vi "Sync_Afterwards.vi"(2 "Analogue Data":dbl[][](array[numeric]) format="%.3f", 4 "LDA Data":dbl[][](array[numeric]) format="%.3f") -> (0 "Eng Values":dbl[][](array[numeric]) format="%.2f")   [LabVIEW 2010]
uses:
  Globals/LDA_meas_global_1.vi
  Globals/Meas_global.vi
  Globals/Dynamic_call_global.ph.vi
panel:
  out "Array":string[](array[string])
  out "Delay (ms)":dbl=13.0 format="%.2f"
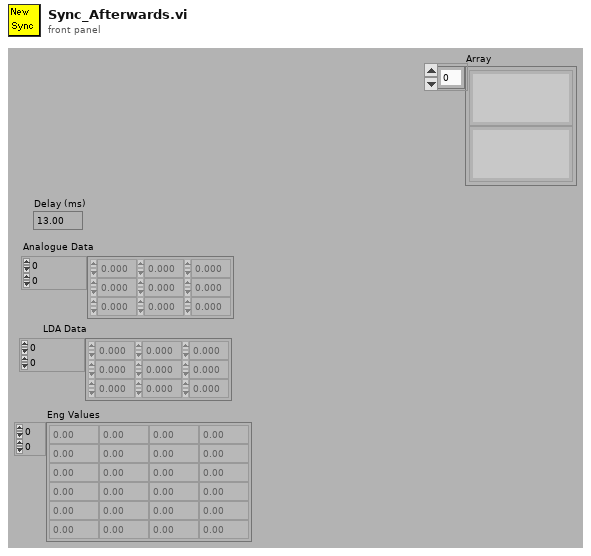
[diagram p1: front panel]
types:
  T1 = typedef "Analysis_info_cluster.ctl" = cluster{"Colour":u32, "Inst type":T2, "Inst name":string, "Symbol":string, "Code name":string, "Extra Info":string, "Inst Array":T3, "Index":i32, "Voltage Index":i32, "Extra Titles":string[], "Extra Values":string[]}
  T2 = typedef "Inst_type.ctl" = enum16{"Propeller anemometer", "Raw voltage", "Pressure Transducer", "Pitot-static tube", "Preston tube", "Hot wire", "Cross wire 1", "Cross wire 2", "Generic Linear", "Generic Polynomial", "Generic BackPoly", "Fast FID", "Thermocouple", "Cold wire", "Pulsed Wire", "LDA Vel", "LDA Tran time", "LDA Arr time"}
  T3 = typedef "Instrument_Array.ctl" = enum16{"PWA", "LDA", "Analogue"}
  T4 = typedef "Analysis_type_cluster.ctl" = cluster{"Analysis type":T5, "Indicies":i32[], "Name":string, "Inst Array":T3, "Info index":i32}
  T5 = typedef "Analysis_type_Enum.ctl" = enum16{"Slow Response", "Fast Response", "Weighted Fast Response", "Fast FID", "Weighted Fast FID", "Cross Wire", "Weighted Cross Wire", "Weighted LDA"}
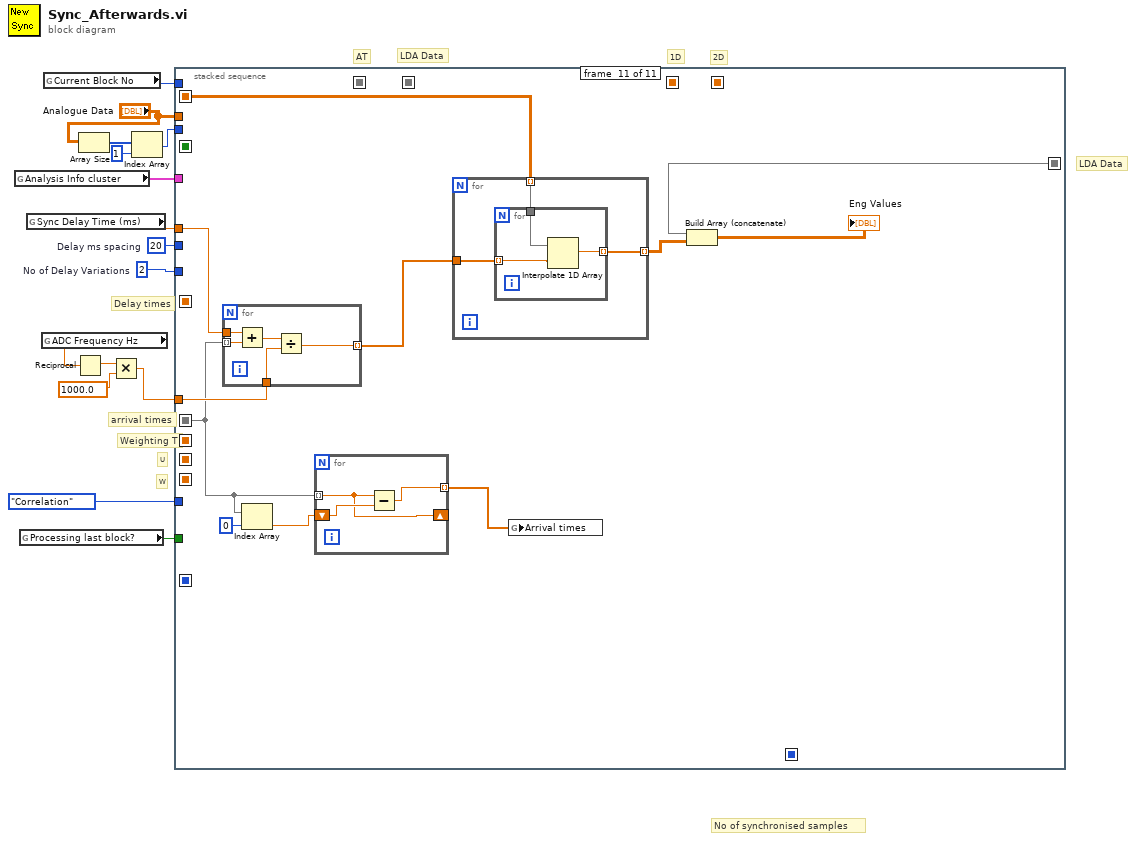
[diagram p0: block diagram]
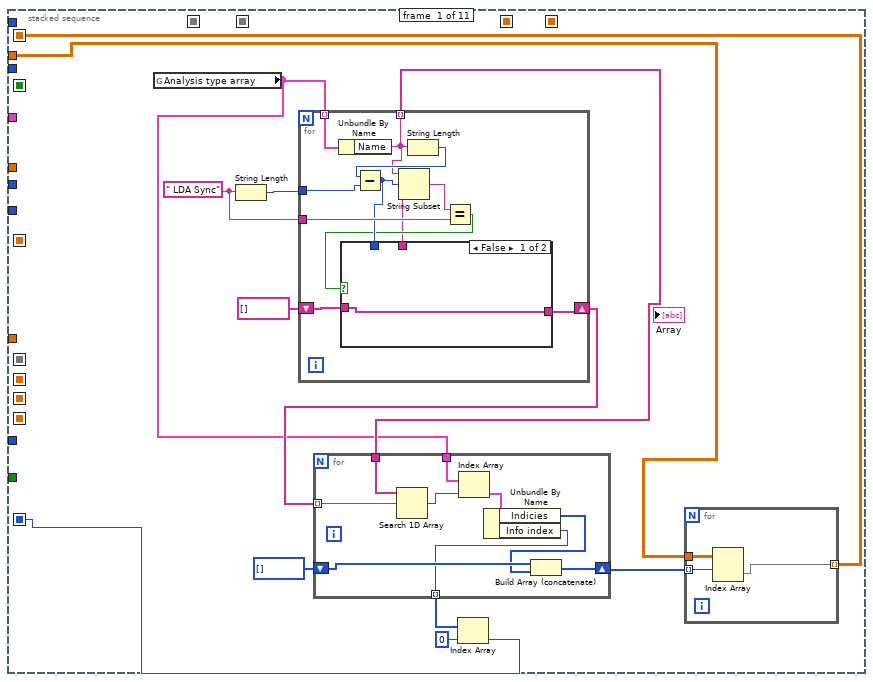
[diagram p2: hidden frame]
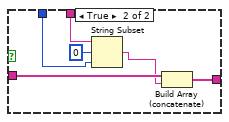
[diagram p3: hidden frame]
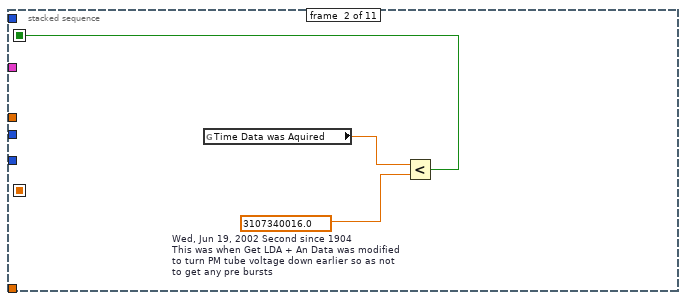
[diagram p4: hidden frame]
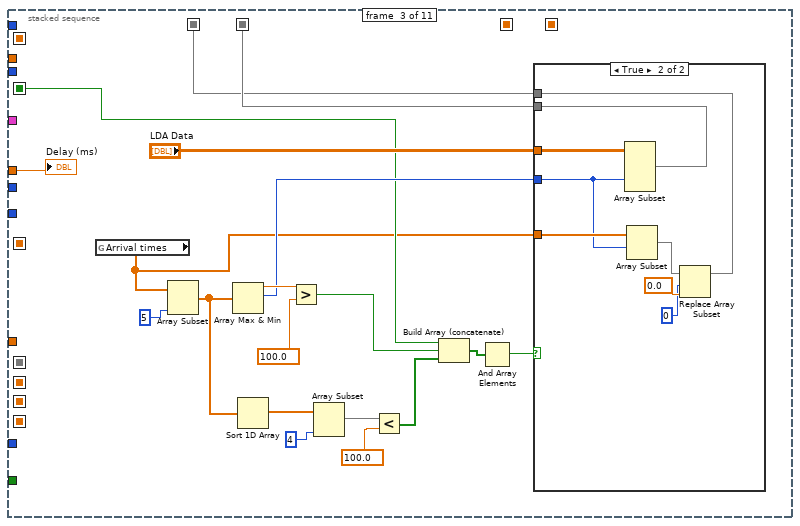
[diagram p5: hidden frame]
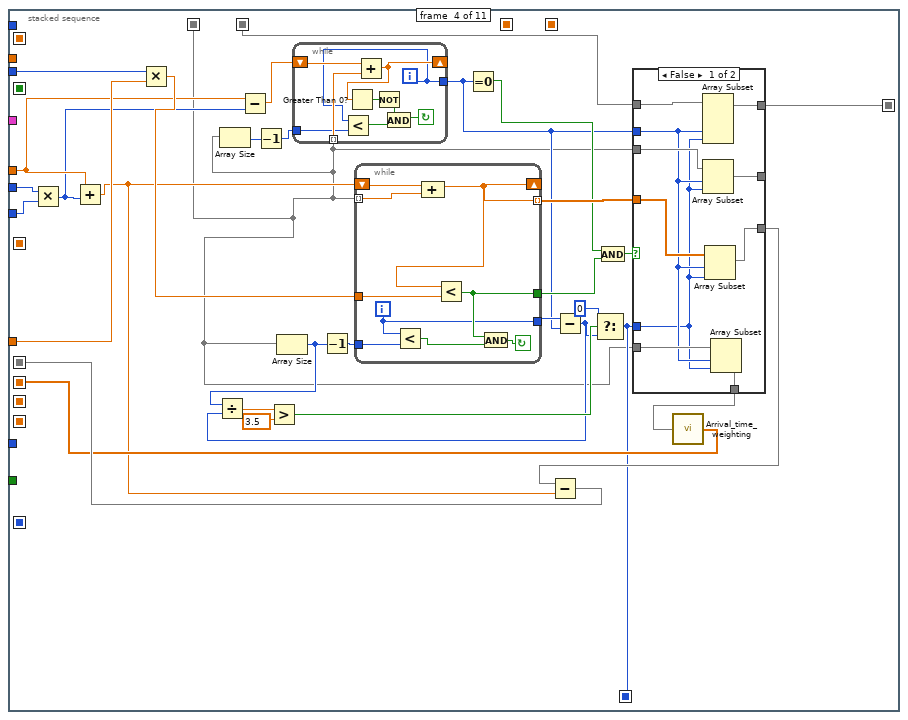
[diagram p7: hidden frame]
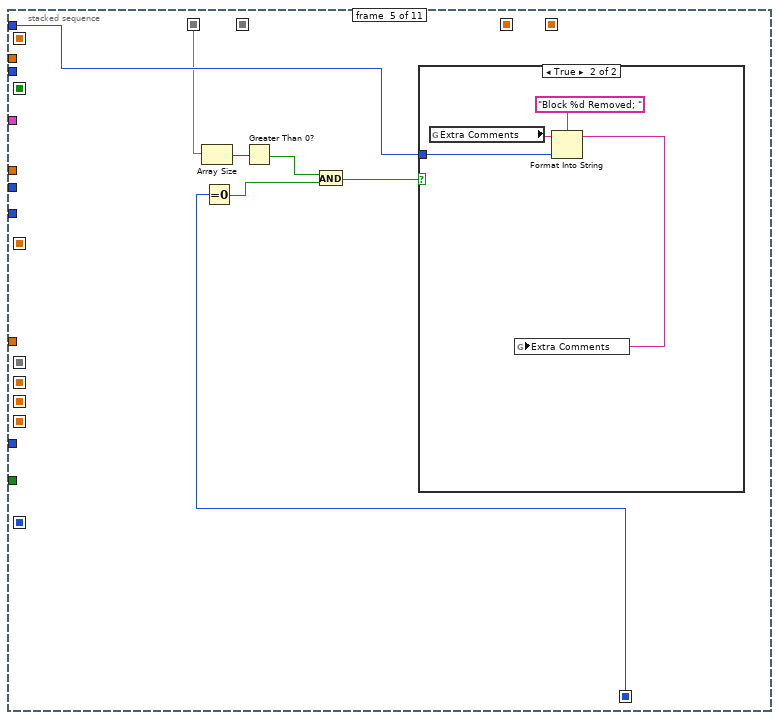
[diagram p9: hidden frame]
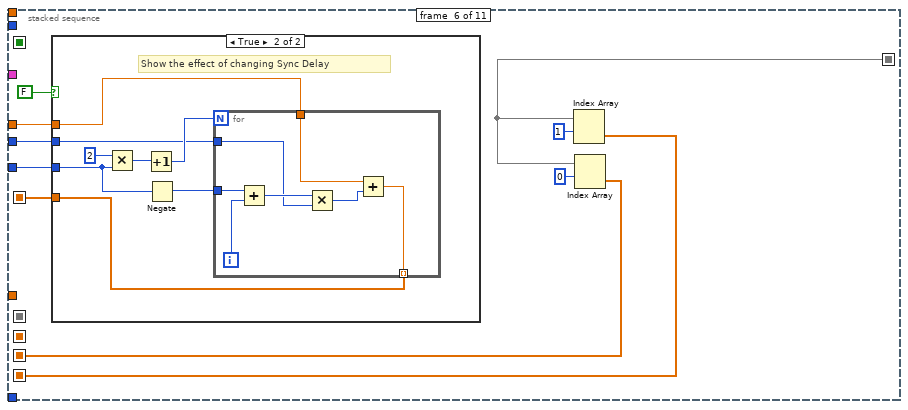
[diagram p11: hidden frame]
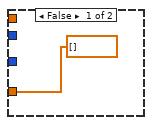
[diagram p12: hidden frame]
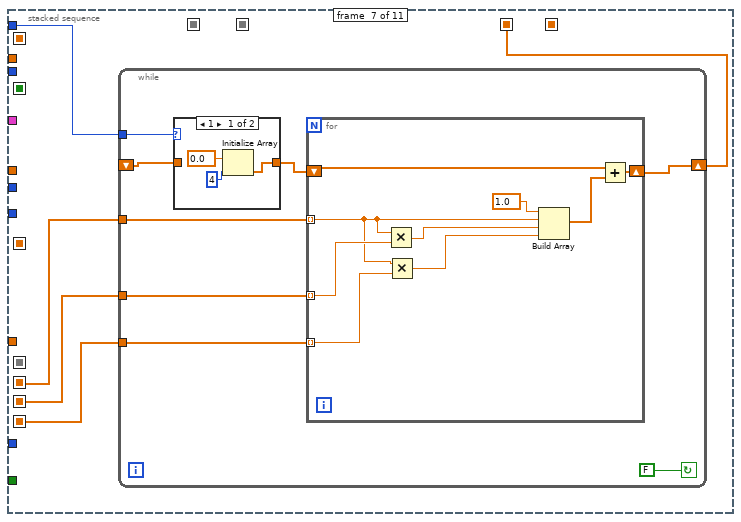
[diagram p13: hidden frame]
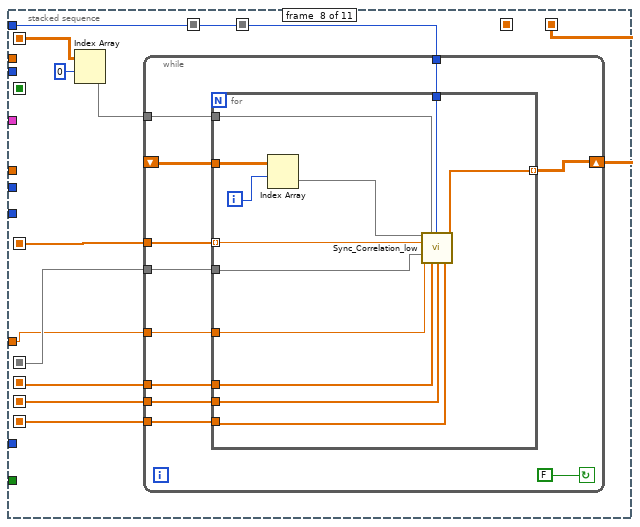
[diagram p15: hidden frame]
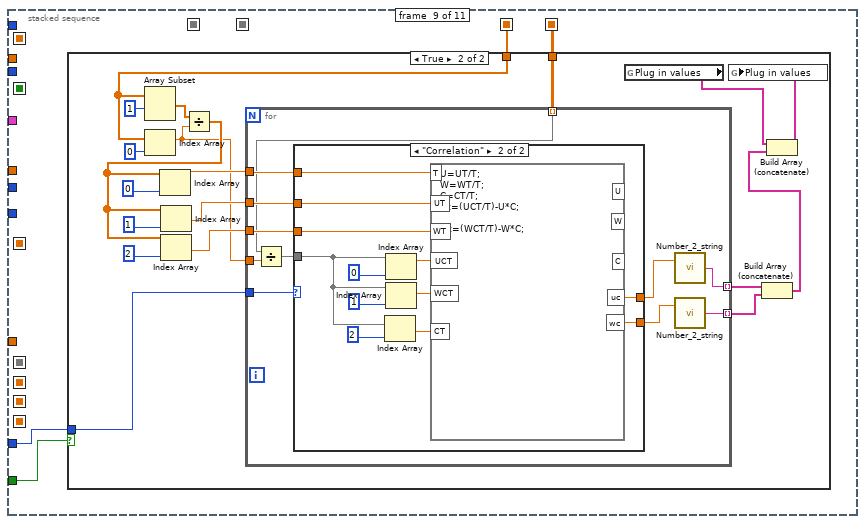
[diagram p16: hidden frame]
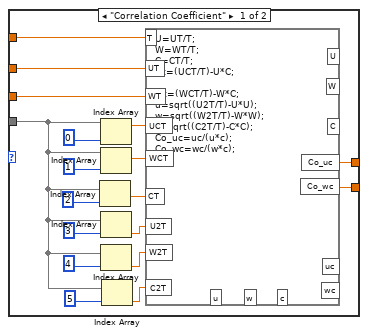
[diagram p18: hidden frame]
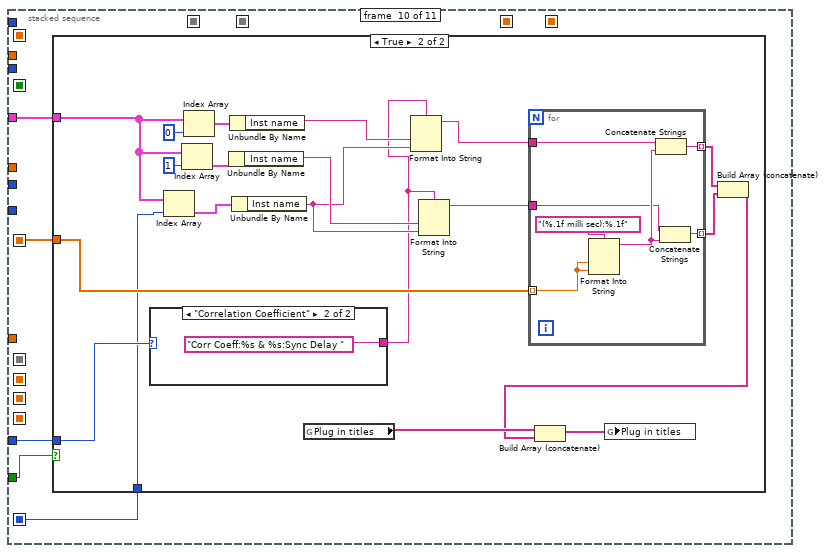
[diagram p19: hidden frame]
diagram:
  w3 = 20  # Delay ms spacing
  w15 = 2  # No of Delay Variations
  # "No of synchronised samples"
  # "AT"
  # "LDA Data"
  # "Delay times"
  # "1D"
  # "2D"
  # "W"
  # "U"
  # "Weighting T"
  # "arrival times"
  # "LDA Data"
  n1 = global read "Meas_global.vi" "Analysis Info cluster"() -> (w1:T1[])
  n2 = global read "Meas_global.vi" "Processing last block?"() -> (w13:bool)
  n3 = global read "LDA_meas_global_1.vi" "Sync Delay Time (ms)"() -> (w8:dbl)
  n4 = global read "LDA_meas_global_1.vi" "ADC Frequency Hz"() -> (w11:dbl)
  n5 = global read "Meas_global.vi" "Current Block No"() -> (w14:i32)
  n6 = Reciprocal(x=w11) -> (1/x=w12:dbl)
  n7 = Array Size(array="Analogue Data") -> (size(s)=w6:i32[])
  n8 = Multiply(x=w12, y=1000.0) -> (x*y=w9:dbl)
  n9 = Index Array(array=w6, index=1 ("Index")) -> (element=w4:i32)
  n10 = stacked-sequence {
    seq-local: [_ _ _ w119 _ _ _ _ _ _ _] -> [_ _ _ _ _ w170 _ _ _ _ w357]
    seq-local: [_ _ _ w116 _ _ _ _ _ _ _] -> [_ _ _ _ _ _ _ w222 _ _ w351]
    seq-local: [_ _ _ w114 _ _ _ _ _ _ _] -> [_ _ _ _ _ _ w195 w223 _ _ _]
    seq-local: [_ _ _ _ _ w169 _ _ _ _ _] -> [_ _ _ _ _ _ w194 w225 _ _ _]
    seq-local: [_ _ _ _ _ w168 _ _ _ _ _] -> [_ _ _ _ _ _ w193 w224 _ _ _]
    seq-local: [_ _ _ _ _ _ _ w220 _ _ _] -> [_ _ _ _ _ _ _ _ w252 _ _]
    seq-local: [_ _ _ _ _ _ w191 _ _ _ _] -> [_ _ _ _ _ _ _ _ w253 _ _]
    seq-local: [_ _ _ _ _ w173 _ _ _ _ _] -> [_ _ _ _ _ _ _ w219 _ w318 _]
    seq-local: [_ _ w66 _ _ _ _ _ _ _ _] -> [_ _ _ w106 _ _ _ _ _ _ _]
    seq-local: [_ _ w65 _ _ _ _ _ _ _ _] -> [_ _ _ w92 w159 _ _ _ _ _ _]
    seq-local: [_ w59 _ _ _ _ _ _ _ _ _] -> [_ _ w62 _ _ _ _ _ _ _ _]
    seq-local: [_ _ _ w96 _ _ _ _ _ _ _] -> [_ _ _ _ w158 _ _ _ _ _ _]
    seq-local: [w17 _ _ _ _ _ _ _ _ _ _] -> [_ _ _ _ _ _ _ _ _ w315 _]
    seq-local: [w16 _ _ _ _ _ _ _ _ _ _] -> [_ _ _ _ _ _ _ w217 _ _ w354]
    tunnel: "Analogue Data" -> [w20 _ _ _ _ _ _ _ _ _ _]
    tunnel: w8 -> [_ _ w63 w108 _ w167 _ _ _ _ w353]
    tunnel: w15 -> [_ _ _ w94 _ w174 _ _ _ _ _]
    tunnel: w14 -> [_ _ _ _ w160 _ w192 w221 _ _ _]
    tunnel: w13 -> [_ _ _ _ _ _ _ _ w254 w319 _]
    tunnel: w9 -> [_ _ _ w113 _ _ _ w218 _ _ w359]
    tunnel: w4 -> [_ _ _ w98 _ _ _ _ _ _ _]
    tunnel: w3 -> [_ _ _ w95 _ w166 _ _ _ _ _]
    tunnel: enum16{"Correlation", "Correlation Coefficient"}."Correlation" -> [_ _ _ _ _ _ _ _ w251 w317 _]
    tunnel: w1 -> [_ _ _ _ _ _ _ _ _ w316 _]
    frame #0 {
      w27 = " LDA Sync" ("Substring")
      n11 = global read "Meas_global.vi" "Analysis type array"() -> (w23:T4[])
      n12 = String Length(string=w27) -> (length=w26:i32)
      n13 = for {
        tunnel: w23 -> [w50] mode=indexing
        tunnel: w26 -> [w48]
        tunnel: w27 -> [w46]
        shift-right: [w42] -> w24
        shift-left: string[] [] -> [w43]
        tunnel: [w41] -> w25 mode=indexing
        n14 = Unbundle By Name(w50) -> ("Name"=w41:string)
        n15 = String Length(string=w41) -> (length=w49:i32)
        n16 = Subtract(x=w49, y=w48) -> (x-y=w45:i32)
        n17 = String Subset(string=w41, offset (0)=w45) -> (substring=w47:string)  [unwired: 1 out]
        n18 = Equal?(x=w47, y=w46) -> (x = y?=w44:bool)
        n19 = case shown="False" w44 {
          tunnel: w41 -> [_ w57]
          tunnel: w45 -> [_ w55]
          tunnel: w43 -> [w51 w54]
          tunnel: [w51 w52] -> w42
          frame False {
          }
          frame True {
            n20 = String Subset(string=w57, offset (0)=0, length (rest)=w55) -> (substring=w53:string)
            n21 = Build Array (concatenate)(w54, w53) -> (w52:string[])
          }
        }
      }
      n22 = for {
        tunnel: w25 -> [w40]
        tunnel: w24 -> [w39] mode=indexing
        tunnel: w23 -> [w38]
        shift-right: [w34] -> w21
        shift-left: i32[] [] -> [w36]
        tunnel: [w32] -> w19 mode=indexing
        n23 = Search 1D Array(1D array=w40, element=w39) -> (index of element=w33:i32)  [unwired: 1 out]
        n24 = Index Array(array=w38, index=w33) -> (element=w37:T4)
        n25 = Unbundle By Name(w37) -> ("Indicies"=w35:i32[], "Info index"=w32:i32)
        n26 = Build Array (concatenate)(w36, w35) -> (w34:i32[])
      }
      n27 = Index Array(array=w19, index=0) -> (element=w17:i32)
      n28 = for {
        tunnel: w21 -> [w31] mode=indexing
        tunnel: w20 -> [w30]
        tunnel: [w29] -> w16 mode=indexing
        n29 = Index Array(array=w30, index (row)=w31) -> (element=w29:dbl[])  [unwired: 1 in]
      }
    }
    frame #1 {
      w60 = 3107340016.0  # Wed, Jun 19, 2002 Second since 1904 This was when Get LDA + An Data was modified to turn PM tube voltage down earlier so as not to get any pre bursts
      n30 = global read "Meas_global.vi" "Time Data was Aquired"() -> (w58:dbl)
      n31 = Less?(x=w58, y=w60) -> (x < y?=w59:bool)
    }
    frame #2 {
      n32 = global read "LDA_meas_global_1.vi" "Arrival times"() -> (w61:dbl[])
      n33 = Array Subset(array=w61, length=5 ("Array Length")) -> (w76:dbl[])  [unwired: 1 in]
      n34 = Array Max & Min(array=w76) -> (max value=w78:dbl, max index (indices)=w68:i32)  [unwired: 2 out]
      n35 = Sort 1D Array(array=w76) -> (sorted array=w74:dbl[])
      n36 = Greater?(x=w78, y=100.0) -> (0:w70:bool)
      n37 = Array Subset(array=w74, length=4 ("Array Length")) -> (w73:dbl[])  [unwired: 1 in]
      n38 = Less?(x=w73, y=100.0) -> (x < y?=w71:bool[])
      n39 = Build Array (concatenate)(w62, w70, w71) -> (w69:bool[])
      n40 = And Array Elements(Boolean array=w69) -> (logical AND=w64:bool)
      n41 = case shown="True" w64 {
        tunnel: w68 -> [_ w82]
        tunnel: "LDA Data" -> [w80 w89]
        tunnel: [w80 w88] -> w66
        tunnel: w61 -> [w81 w87]
        tunnel: [w81 w83] -> w65
        frame False {
        }
        frame True {
          n42 = Array Subset(array=w89, index (col)=w82) -> (w88:dbl[][])  [unwired: 3 in]
          n43 = Array Subset(array=w87, index=w82) -> (w86:dbl[])  [unwired: 1 in]
          n44 = Replace Array Subset(array=w86, new element=0.0 ("Element Data"), index=0 ("Index")) -> (w83:dbl[])
        }
      }
      "Delay (ms)" <- w63
    }
    frame #3 {
      n45 = Multiply(x=w95, y=w94) -> (x*y=w93:i32)
      n46 = Add(x=w108, y=w93) -> (x+y=w112:dbl)
      n47 = Multiply(x=w98, y=w113) -> (x*y=w120:dbl)
      n48 = Array Size(array=w92) -> (size(s)=w91:i32)
      n49 = Subtract(x=w108, y=w93) -> (x-y=w107:dbl)
      n50 = Decrement(x=w91) -> (x-1=w90:i32)
      n51 = Array Size(array=w92) -> (size(s)=w101:i32)
      n52 = while {
        tunnel: [w132] -> w104
        tunnel: w92 -> [w134] mode=indexing
        shift-left: w107 -> [w139]
        shift-right: [w138] -> _
        tunnel: w90 -> [w131]
        i -> [w132]
        stop <- w135 continue-if-true
        n53 = Less?(x=w132, y=w131) -> (x < y?=w133:bool)
        n54 = Add(x=w139, y=w134) -> (x+y=w138:dbl)
        n55 = Greater Than 0?(x=w138) -> (x > 0?=w137:bool)
        n56 = Not(x=w137) -> (.not. x?=w136:bool)
        n57 = And(x=w136, y=w133) -> (x .and. y?=w135:bool)
      }
      n58 = Decrement(x=w101) -> (x-1=w121:i32)
      n59 = while {
        tunnel: [w122] -> w118 mode=indexing
        tunnel: [w123] -> w105
        tunnel: [w124] -> w111
        tunnel: w120 -> [w127]
        tunnel: w121 -> [w128]
        tunnel: w92 -> [w129] mode=indexing
        shift-left: w112 -> [w130]
        shift-right: [w122] -> _
        i -> [w123]
        stop <- w125 continue-if-true
        n60 = Less?(x=w123, y=w128) -> (x < y?=w126:bool)
        n61 = Compound Arithmetic op=ADD(w130, w129) -> (w122:dbl)
        n62 = Less?(x=w122, y=w127) -> (x < y?=w124:bool)
        n63 = And(x=w124, y=w126) -> (x .and. y?=w125:bool)
      }
      n64 = Equal To 0?(x=w104) -> (x = 0?=w110:bool)
      n65 = Subtract(x=w105, y=w104) -> (x-y=w97:i32)
      n66 = Divide(x=w101, y=w97) -> (x/y=w102:dbl)
      n67 = Greater?(x=w102, y=3.5) -> (0:w100:bool)
      n68 = Select(t=0, s=w100, f=w97) -> (s? t:f=w96:i32)
      n69 = And(x=w110, y=w111) -> (x .and. y?=w109:bool)
      n70 = case shown="False" w109 {
        tunnel: [w149 w152] -> w117
        tunnel: w96 -> [w141 _]
        tunnel: w106 -> [w148 w153]
        tunnel: [w147 w153] -> w119
        tunnel: w118 -> [w146 w152]
        tunnel: w92 -> [w145 w151]
        tunnel: [w144 w151] -> w115
        tunnel: w104 -> [w142 _]
        tunnel: w92 -> [w143 w150]
        tunnel: [w140 w150] -> _
        frame False {
          n71 = Array Subset(array=w148, index (col)=w142, length (col)=w141) -> (w147:dbl[][])  [unwired: 2 in]
          n72 = Array Subset(array=w143, index=w142, length=w141) -> (w140:dbl[])
          n73 = Array Subset(array=w146, index=w142, length=w141) -> (w149:dbl[])
          n74 = Array Subset(array=w145, index=w142, length=w141) -> (w144:dbl[])
        }
        frame True {
        }
      }
      n75 = Subtract(x=w117, y=w112) -> (x-y=w116:dbl[])
      n76 = call "Arrival_time_weighting.vi"("Arrival times"=w115) -> ("Weighting"=w114:dbl[])
    }
    frame #4 {
      n77 = Array Size(array=w159) -> (size(s)=w157:i32)
      n78 = Equal To 0?(x=w158) -> (x = 0?=w155:bool)
      n79 = Greater Than 0?(x=w157) -> (x > 0?=w156:bool)
      n80 = And(x=w156, y=w155) -> (x .and. y?=w154:bool)
      n81 = case shown="True" w154 {
        tunnel: w160 -> [_ w164]
        frame False {
        }
        frame True {
          n82 = global read "Meas_global.vi" "Extra Comments"() -> (w162:string)
          n83 = Format Into String(format string="Block %d Removed; " ("Format String"), initial string=w162, w164) -> (resulting string=w161:string)  [unwired: 1 in, 1 out]
          n84 = global write "Meas_global.vi" "Extra Comments"(w161) -> ()
        }
      }
    }
    frame #5 {
      n85 = case shown="True" FALSE {
        tunnel: w174 -> [_ w180]
        tunnel: [dbl[] [] w178] -> w173
        tunnel: w167 -> [_ w177]
        tunnel: w166 -> [_ w176]
        frame False {
        }
        frame True {
          # "Show the effect of changing Sync Delay"
          n86 = Multiply(x=2, y=w180) -> (x*y=w182:i32)
          n87 = Increment(x=w182) -> (x+1=w181:i32)
          n88 = Negate(x=w180) -> (-x=w179:i32)
          n89 = for {
            N: w181 -> [_]
            tunnel: w179 -> [w190]
            tunnel: w177 -> [w188]
            tunnel: [w187] -> w178 mode=indexing
            tunnel: w176 -> [w184]
            i -> [w189]
            n90 = Add(x=w190, y=w189) -> (x+y=w186:i32)
            n91 = Multiply(x=w186, y=w184) -> (x*y=w185:i32)
            n92 = Add(x=w188, y=w185) -> (x+y=w187:dbl)
          }
        }
      }
      n93 = Index Array(array=w170, index (row)=1 ("Index")) -> (element=w168:dbl[])  [unwired: 1 in]
      n94 = Index Array(array=w170, index (row)=0 ("Index")) -> (element=w169:dbl[])  [unwired: 1 in]
    }
    frame #6 {
      n95 = while {
        tunnel: w192 -> [w197]
        tunnel: w193 -> [w201]
        tunnel: w194 -> [w202]
        tunnel: w195 -> [w203]
        shift-left: _ -> [w199]
        shift-right: [w198] -> w191
        stop <- FALSE continue-if-true
        n96 = case shown="1" w197 {
          tunnel: [w204 w207] -> w200
          tunnel: w199 -> [_ w207]
          frame 1 {
            n97 = Initialize Array(0.0 ("Element Data"), 4 ("Dimension Size")) -> (w204:dbl[])
          }
          frame 2, Default {
          }
        }
        n98 = for {
          shift-right: [w215] -> w198
          shift-left: w200 -> [w216]
          tunnel: w203 -> [w211] mode=indexing
          tunnel: w202 -> [w214] mode=indexing
          tunnel: w201 -> [w210] mode=indexing
          n99 = Multiply(x=w211, y=w214) -> (x*y=w213:dbl)
          n100 = Multiply(x=w211, y=w210) -> (x*y=w209:dbl)
          n101 = Build Array(1.0 ("Input Element"), w211, w213, w209) -> (w208:dbl[])
          n102 = Add(x=w216, y=w208) -> (x+y=w215:dbl[])
        }
      }
    }
    frame #7 {
      n103 = Index Array(array=w217, index (row)=0 ("Index")) -> (element=w226:dbl[])  [unwired: 1 in]
      n104 = while {
        tunnel: w219 -> [w229]
        shift-left: _ -> [w231]
        shift-right: [w230] -> w220
        tunnel: w221 -> [w232]
        tunnel: w222 -> [w233]
        tunnel: w223 -> [w234]
        tunnel: w224 -> [w235]
        tunnel: w225 -> [w236]
        tunnel: w226 -> [w237]
        tunnel: w218 -> [w238]
        stop <- FALSE continue-if-true
        n105 = for {
          tunnel: w233 -> [w250]
          tunnel: w238 -> [w249]
          tunnel: w237 -> [w248]
          tunnel: w236 -> [w247]
          tunnel: w235 -> [w246]
          tunnel: w234 -> [w245]
          tunnel: [w244] -> w230 mode=indexing
          tunnel: w232 -> [w243]
          tunnel: w231 -> [w241]
          tunnel: w229 -> [w239] mode=indexing
          i -> [w240]
          n106 = Index Array(array=w241, index (row)=w240) -> (element=w242:dbl[])  [unwired: 1 in]
          n107 = call "Sync_Correlation_low.vi"("Shift In"=w242, "Analogue Data"=w248, "Block No"=w243, "Delay (ms)"=w239, "Arrival Times"=w250, "Delta T (ms)"=w249, "T"=w245, "U"=w247, "W"=w246) -> ("Shift Out"=w244:dbl[])  [unwired: 6 out]
        }
      }
    }
    frame #8 {
      n108 = case shown="True" w254 {
        tunnel: w253 -> [_ w271]
        tunnel: w252 -> [_ w261]
        tunnel: w251 -> [_ w259]
        frame False {
        }
        frame True {
          n109 = Array Subset(array=w271, index=1 ("Array Index")) -> (w270:dbl[])  [unwired: 1 in]
          n110 = Index Array(array=w271, index=0 ("Index")) -> (element=w262:dbl)
          n111 = Divide(x=w270, y=w262) -> (x/y=w266:dbl[])
          n112 = Index Array(array=w266, index=0) -> (element=w265:dbl)
          n113 = Index Array(array=w266, index=1) -> (element=w264:dbl)
          n114 = Index Array(array=w266, index=2) -> (element=w263:dbl)
          n115 = for {
            tunnel: w265 -> [w282]
            tunnel: w264 -> [w284]
            tunnel: w263 -> [w283]
            tunnel: w262 -> [w281]
            tunnel: w261 -> [w280] mode=indexing
            tunnel: w259 -> [w278]
            tunnel: [w275] -> w257 mode=indexing
            tunnel: [w274] -> w256 mode=indexing
            n116 = Divide(x=w280, y=w281) -> (x/y=w279:dbl[])
            n117 = case shown="\"Correlation\"" w278 {
              tunnel: w284 -> [w299 w311]
              tunnel: w283 -> [w298 w310]
              tunnel: w282 -> [w294 w306]
              tunnel: w279 -> [w290 w305]
              tunnel: [w286 w304] -> w277
              tunnel: [w285 w303] -> w276
              frame "Correlation Coefficient" {
                n118 = Index Array(array=w290, index=2) -> (element=w295:dbl)
                n119 = Index Array(array=w290, index=0) -> (element=w297:dbl)
                n120 = Index Array(array=w290, index=1) -> (element=w296:dbl)
                n121 = Index Array(array=w290, index=3) -> (element=w287:dbl)
                n122 = Index Array(array=w290, index=4) -> (element=w288:dbl)
                n123 = Index Array(array=w290, index=5) -> (element=w289:dbl)
                n124 = formula code="U=UT/T;\nW=WT/T;\nC=CT/T;\nuc=(UCT/T)-U*C;\n\nwc=(WCT/T)-W*C;\nu=sqrt((U2T/T)-U*U);\nw=sqrt((W2T/T)-W*W);\nc=sqrt((C2T/T)-C*C);\nCo_uc=uc/(u*c);\nCo_wc=wc/(w*c);"("T"=w294, "UT"=w299, "WT"=w298, "WCT"=w296, "CT"=w295, "UCT"=w297, "U2T"=w287, "W2T"=w288, "C2T"=w289) -> ("Co_uc"=w286:dbl, "Co_wc"=w285:dbl)  [unwired: 8 out]
              }
              frame "Correlation" {
                n125 = Index Array(array=w305, index=2) -> (element=w307:dbl)
                n126 = Index Array(array=w305, index=0) -> (element=w309:dbl)
                n127 = Index Array(array=w305, index=1) -> (element=w308:dbl)
                n128 = formula code="U=UT/T;\nW=WT/T;\nC=CT/T;\nuc=(UCT/T)-U*C;\n\nwc=(WCT/T)-W*C;"("T"=w306, "UT"=w311, "WT"=w310, "WCT"=w308, "CT"=w307, "UCT"=w309) -> ("uc"=w304:dbl, "wc"=w303:dbl)  [unwired: 3 out]
              }
            }
            n129 = call "Number_2_string.vi"("number"=w277) -> ("String"=w274:string)  [unwired: 1 in]
            n130 = call "Number_2_string.vi"("number"=w276) -> ("String"=w275:string)  [unwired: 1 in]
          }
          n131 = global read "Dynamic_call_global.ph.vi" "Plug in values"() -> (w258:string[])
          n132 = Build Array (concatenate)(w256, w257) -> (w255:string[])
          n133 = Build Array (concatenate)(w258, w255) -> (w260:string[])
          n134 = global write "Dynamic_call_global.ph.vi" "Plug in values"(w260) -> ()
        }
      }
    }
    frame #9 {
      n135 = case shown="True" w319 {
        tunnel: w318 -> [_ w332]
        tunnel: w317 -> [_ w323]
        tunnel: w316 -> [_ w321]
        tunnel: w315 -> [_ w320]
        frame False {
        }
        frame True {
          n136 = case shown="\"Correlation Coefficient\"" w323 {
            tunnel: ["Correlation:%s & %s:Sync Delay " ("Format String") "Corr Coeff:%s & %s:Sync Delay " ("Format String")] -> w322
            frame "Correlation" {
            }
            frame "Correlation Coefficient" {
            }
          }
          n137 = Index Array(array=w321, index=w320) -> (element=w337:T1)
          n138 = Index Array(array=w321, index=1 ("Index")) -> (element=w333:T1)
          n139 = Index Array(array=w321, index=0 ("Index")) -> (element=w334:T1)
          n140 = Unbundle By Name(w333) -> ("Inst name"=w330:string)
          n141 = Unbundle By Name(w334) -> ("Inst name"=w331:string)
          n142 = Unbundle By Name(w337) -> ("Inst name"=w329:string)
          n143 = global read "Dynamic_call_global.ph.vi" "Plug in titles"() -> (w339:string[])
          n144 = Format Into String(format string=w322, w331, w329) -> (resulting string=w328:string)  [unwired: 2 in, 1 out]
          n145 = Format Into String(format string=w322, w330, w329) -> (resulting string=w327:string)  [unwired: 2 in, 1 out]
          n146 = for {
            tunnel: w332 -> [w347] mode=indexing
            tunnel: w328 -> [w345]
            tunnel: w327 -> [w344]
            tunnel: [w343] -> w326 mode=indexing
            tunnel: [w342] -> w325 mode=indexing
            n147 = Format Into String(format string="(%.1f milli sec):%.1f" ("Format String"), w347, w347) -> (resulting string=w346:string)  [unwired: 2 in, 1 out]
            n148 = Concatenate Strings(w345, w346) -> (w343:string)
            n149 = Concatenate Strings(w344, w346) -> (w342:string)
          }
          n150 = Build Array (concatenate)(w326, w325) -> (w324:string[])
          n151 = Build Array (concatenate)(w339, w324) -> (w338:string[])
          n152 = global write "Dynamic_call_global.ph.vi" "Plug in titles"(w338) -> ()
        }
      }
    }
    frame #10 {
      n153 = for {
        tunnel: w353 -> [w367]
        tunnel: w351 -> [w366] mode=indexing
        tunnel: w359 -> [w365]
        tunnel: [w364] -> w358 mode=indexing
        n154 = Add(x=w367, y=w366) -> (x+y=w363:dbl)
        n155 = Divide(x=w363, y=w365) -> (x/y=w364:dbl)
      }
      n156 = Index Array(array=w351, index=0) -> (element=w349:dbl)
      n157 = for {
        shift-right: [w360] -> _
        shift-left: w349 -> [w362]
        tunnel: w351 -> [w360] mode=indexing
        tunnel: [w361] -> w352 mode=indexing
        n158 = Subtract(x=w360, y=w362) -> (x-y=w361:dbl)
      }
      n159 = for {
        tunnel: w354 -> [w370] mode=indexing
        tunnel: w358 -> [w369]
        tunnel: [w368] -> w356 mode=indexing
        n160 = for {
          tunnel: w370 -> [w373]
          tunnel: w369 -> [w372] mode=indexing
          tunnel: [w371] -> w368 mode=indexing
          n161 = Interpolate 1D Array(1:w372, 2:w373) -> (0:w371:dbl)
        }
      }
      n162 = global write "LDA_meas_global_1.vi" "Arrival times"(w352) -> ()
      n163 = Build Array (concatenate)(w357, w356) -> (→"Eng Values":dbl[][])
    }
  }
